vi "Write Collision state.vi"(10 "Collision state":bool, 11 "Collision in":refnum<class "Collision.lvclass">) -> (3 "Collision out":refnum<class "Collision.lvclass">)   [LabVIEW 2024, in "Collision.lvclass"]
doc: "MIT Licence\nCopyright (c) 2024 David Grollier"
uses:
  Collision.lvclass
  Collision.lvclass/Collision.ctl
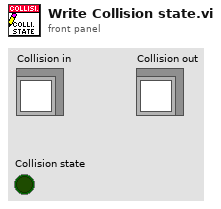
[diagram p1: front panel]
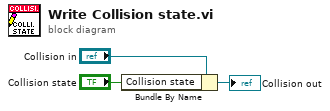
[diagram p0: block diagram]
diagram:
  n1 = Bundle By Name(cluster="Collision in", "Collision state"="Collision state") -> (→"Collision out":refnum<class "Collision.lvclass">)
